vi "Init.vi"(5 "PathControl.lvclass":refnum<class "PathControl.lvclass">, 6 "Environmental classes":refnum<class "Instrument.lvclass">[](array[class]), 7 "XML Handler.lvclass":refnum<class "XML Handler.lvclass">, 8 "error in (no error)":errorcluster, 9 "Instrumentes to Use":T1(array[cluster]), 10 "Device.lvclass":refnum<class "Device.lvclass">, 11 "MCCW ACLR in":refnum<class "MCCW ACLR.lvclass">) -> (0 "error out":errorcluster, 3 "MCCW ACLR out":refnum<class "MCCW ACLR.lvclass">)   [LabVIEW 2020, in "MCCW ACLR.lvclass"]
doc: "Initializes the measurement.\nThis verifies that the instruments are present and adds them into the class data.\nIs also adds the xml handler into the class data."
uses:
  MCCW ACLR.lvclass
  C:/Sandbox/Git_Sandbox/WiSpry Test Framework source code (LV20)/WiSpry Test Framework/Measurements/Measurement.lvclass
  Devices/Device.lvclass
  Instruments/Instrument.lvclass
  XML Handler/XML Handler.lvclass
  Path Control/PathControl.lvclass
  Controls/Init States.ctl
  Instruments/Vector Signal Generator/Vector Signal Generator.lvclass
  Instruments/Spectrum Analyzer/Spectrum Analyzer.lvclass
  MCCW ACLR.lvclass/MCCW ACLR.ctl
  Measurement.lvclass/Measurement.ctl
  Devices/Controls/Change setting mode enum.ctl
  Path Control/Measurements Specific Paths.ctl
  Measurement.lvclass
  Devices/PIC-device/PIC-Device.lvclass
panel:
  out "Current State":string
  out "Initializing MCCW ACLR Measurement":u8(slide) scale=0.0..100.0
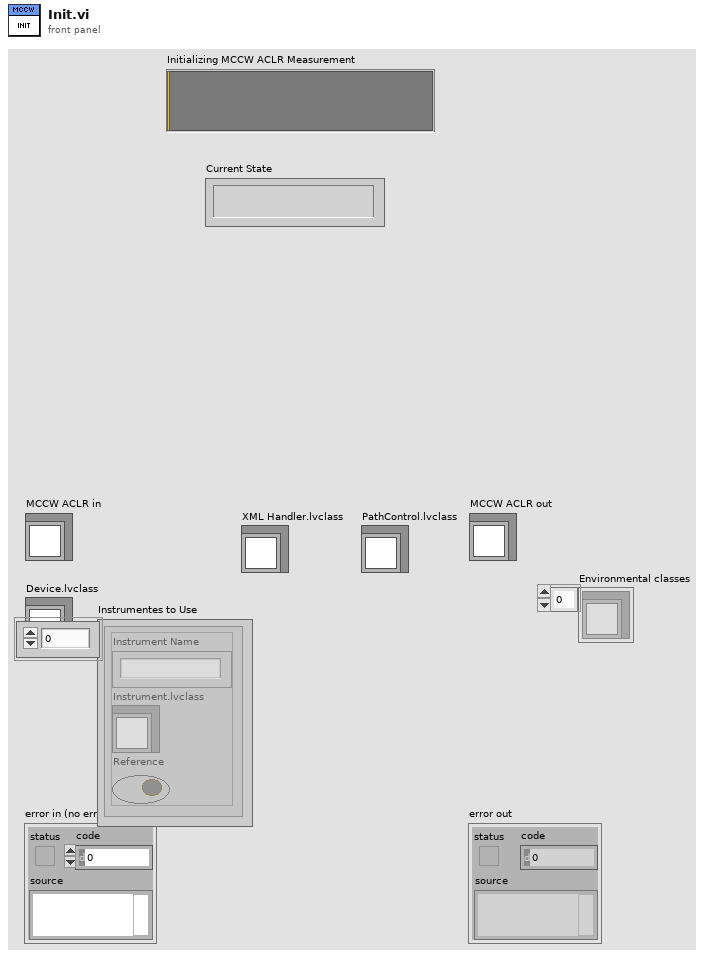
[diagram p1: front panel]
types:
  T1 = cluster{"Instrument Name":string, "Instrument.lvclass":refnum<class "Instrument.lvclass">, "Reference":bool}[]
  T2 = typedef "Measurement.lvclass/Init States.ctl" = enum16{"Verify instruments", "Init Parameters", "Init Instruments", "Add Device", "Init Device", "Create test in XML", "Set path", "Done"}
  T3 = cluster{"List":dbl[], "Index":i32, "Last":bool, "BW [MHz]":dbl}
  T4 = cluster{"Number of Measurements":u32, "Current Measurement":u32, "Last":bool}
  T5 = enum16{"ACLR Configuration", "Reference Level", "Both"}
  T6 = typedef "PIC-Device.lvclass/Change setting mode enum.ctl" = enum16{"Init", "Next", "Reset"}
  T7 = typedef "PathControl.lvclass/Measurements Specific Paths.ctl" = enum16{"No calibration", "Harmonics", "IMD", "S Parameter", "AM-AM", "MCCW-ACLR", "DC", "LCR", "Power Meter GUI", "RF Power"}
  T8 = typedef "MCCW ACLR.lvclass/ACLR configuration.ctl" = cluster{"Frequency":cluster{"Cluster ":cluster{"From":dbl, "To":dbl, "Step":dbl}, "Array":dbl[], "Use Array":bool}, "Power":cluster{"Cluster ":cluster{"From":dbl, "To":dbl, "Step":dbl}, "Array":dbl[], "Use Array":bool}, "Carriers":cluster{"Cluster ":cluster{"From":dbl, "To":dbl, "Step":dbl}, "Array":dbl[], "Use Array":bool}, "Phase Value":dbl, "Number of Measurements":u32, "Use random phase":bool, "Signal BW [MHz] ":dbl}
  T9 = cluster{"Cluster ":cluster{"From":dbl, "To":dbl, "Step":dbl}, "Array":dbl[], "Use Array":bool}
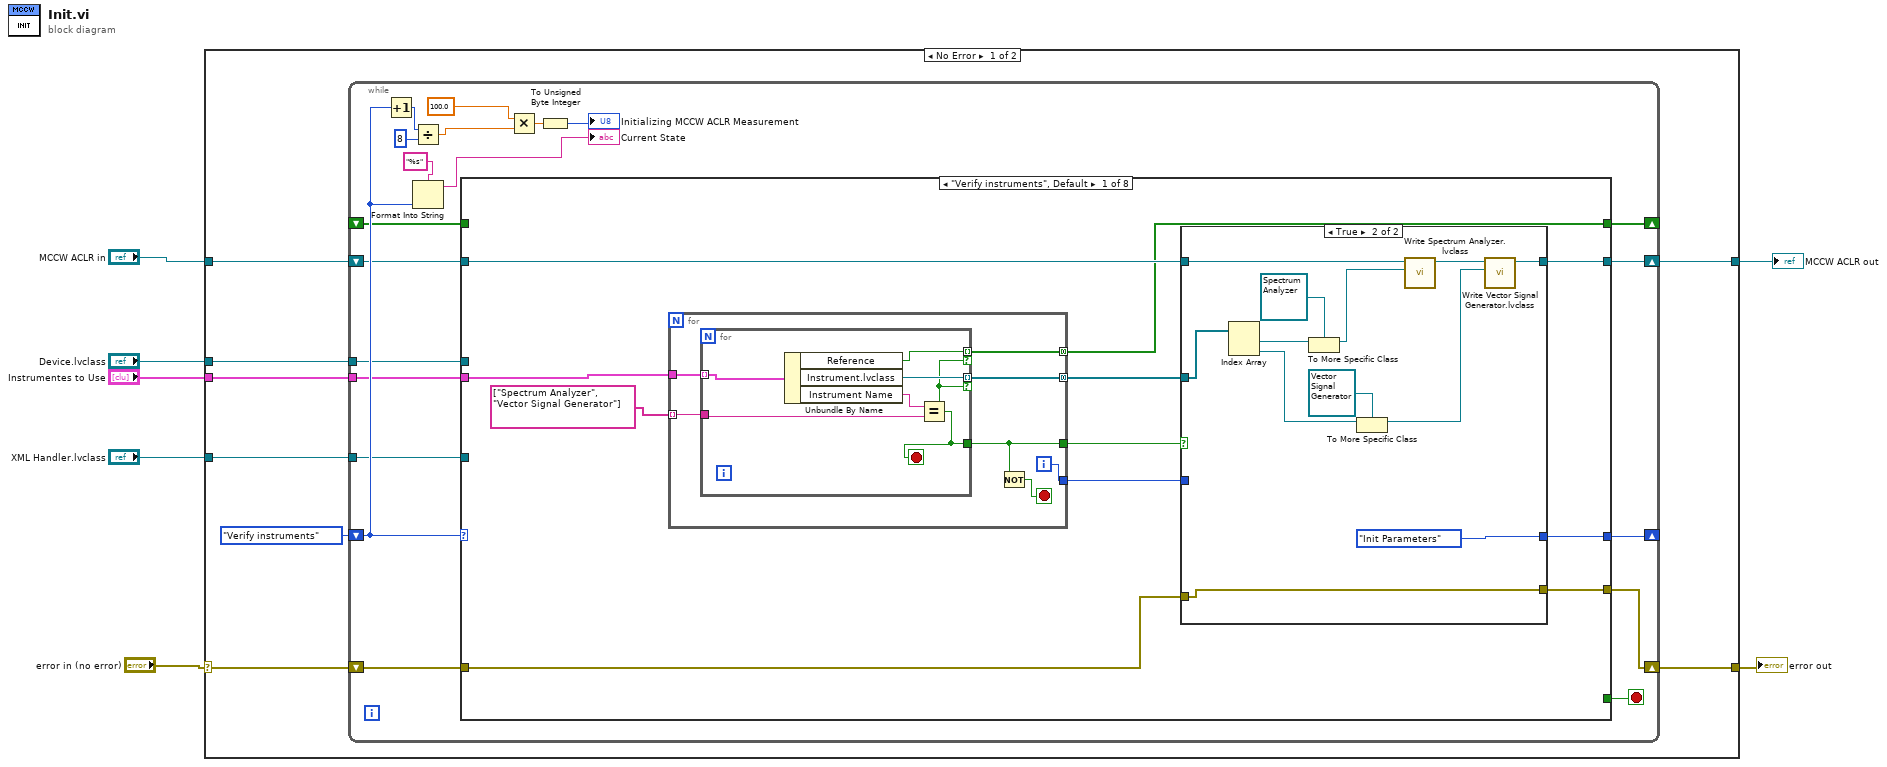
[diagram p0: block diagram]
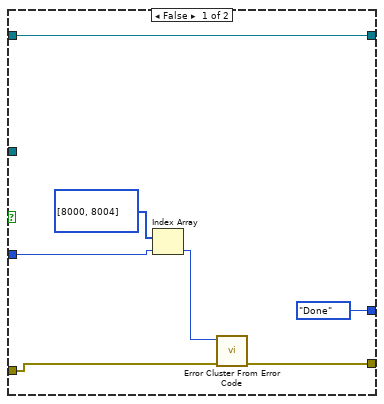
[diagram p2: hidden frame]
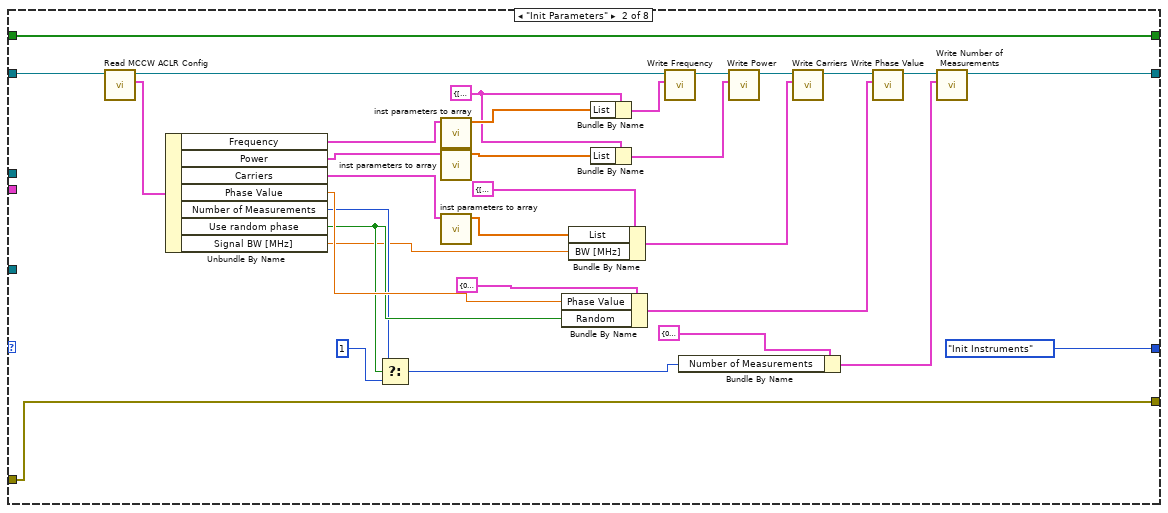
[diagram p3: hidden frame]
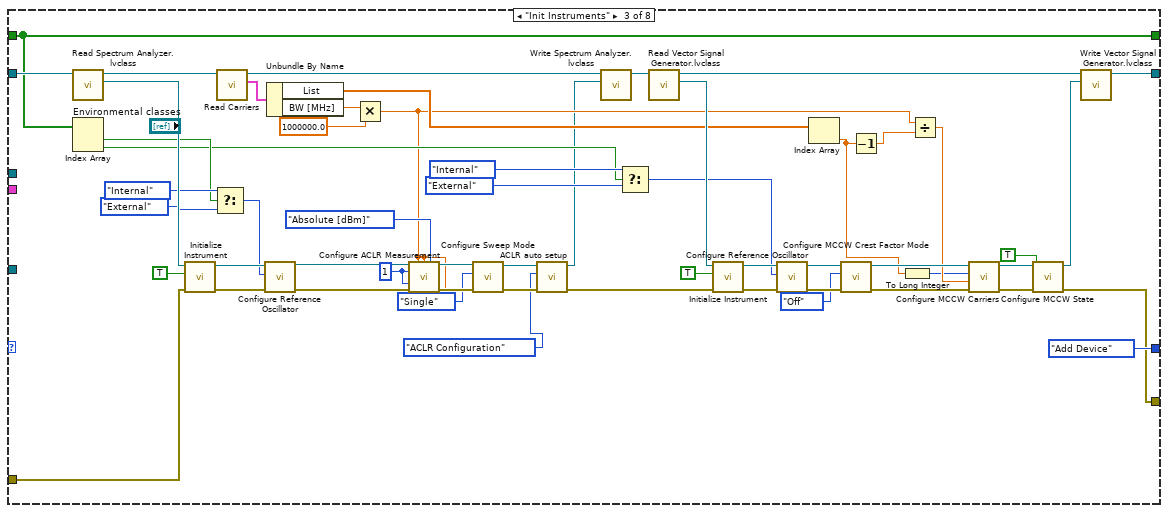
[diagram p4: hidden frame]
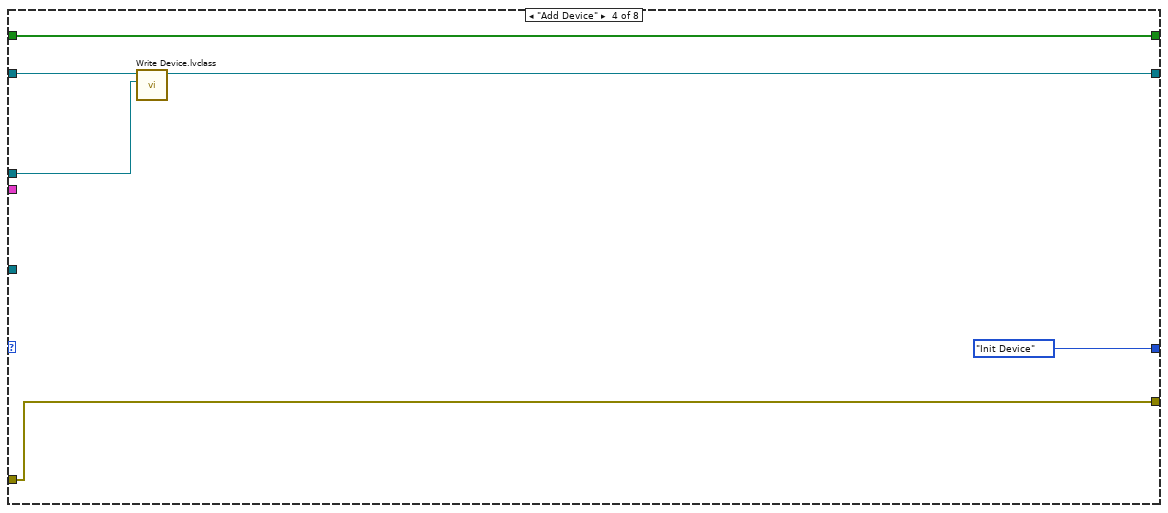
[diagram p5: hidden frame]
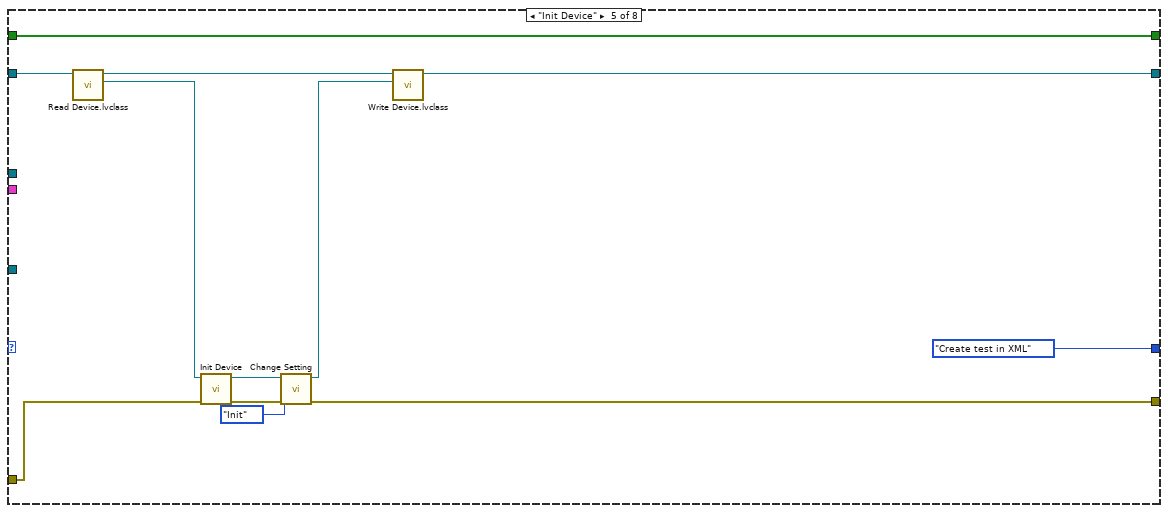
[diagram p6: hidden frame]
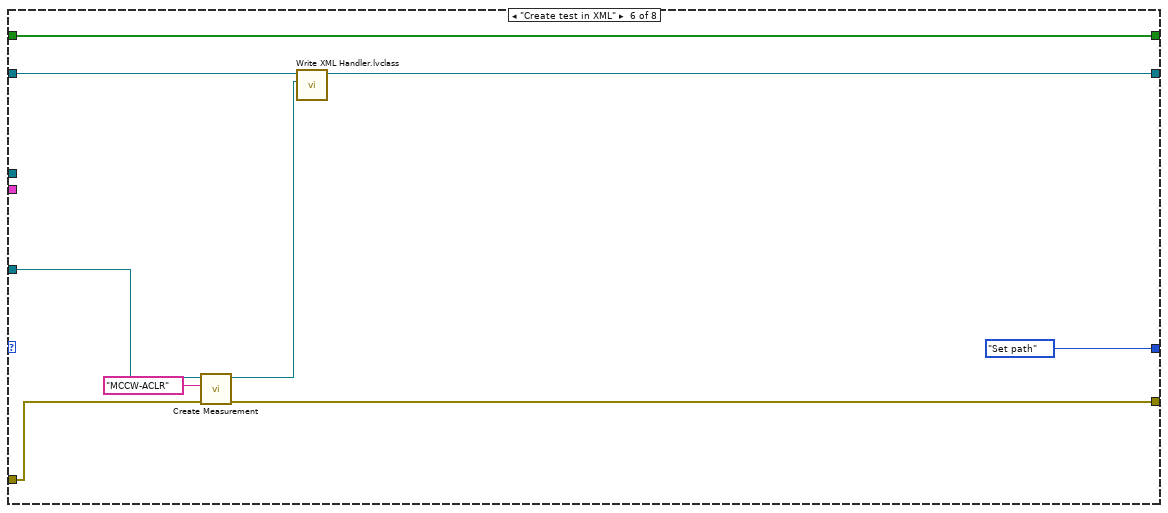
[diagram p7: hidden frame]
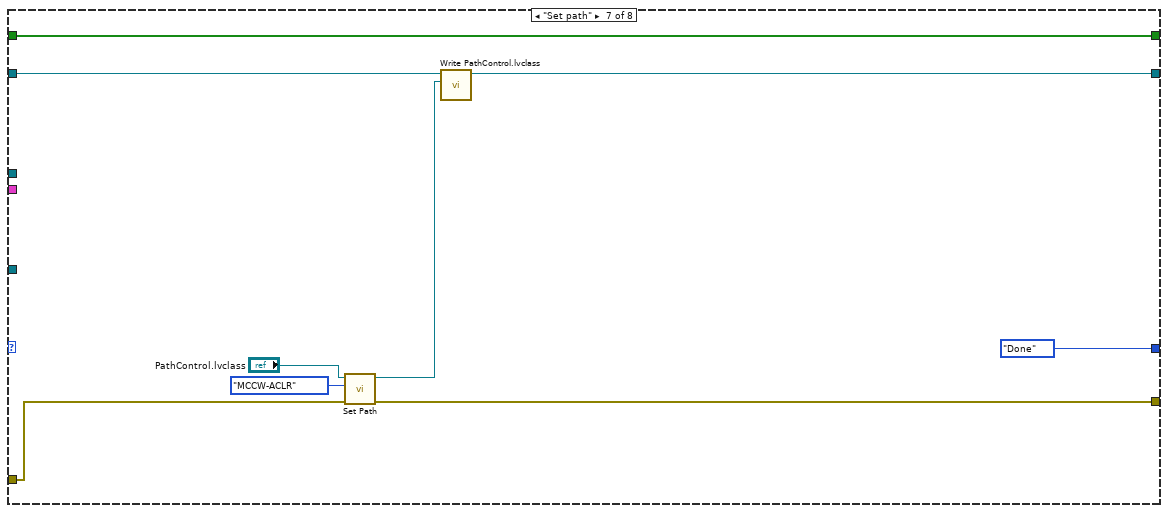
[diagram p8: hidden frame]
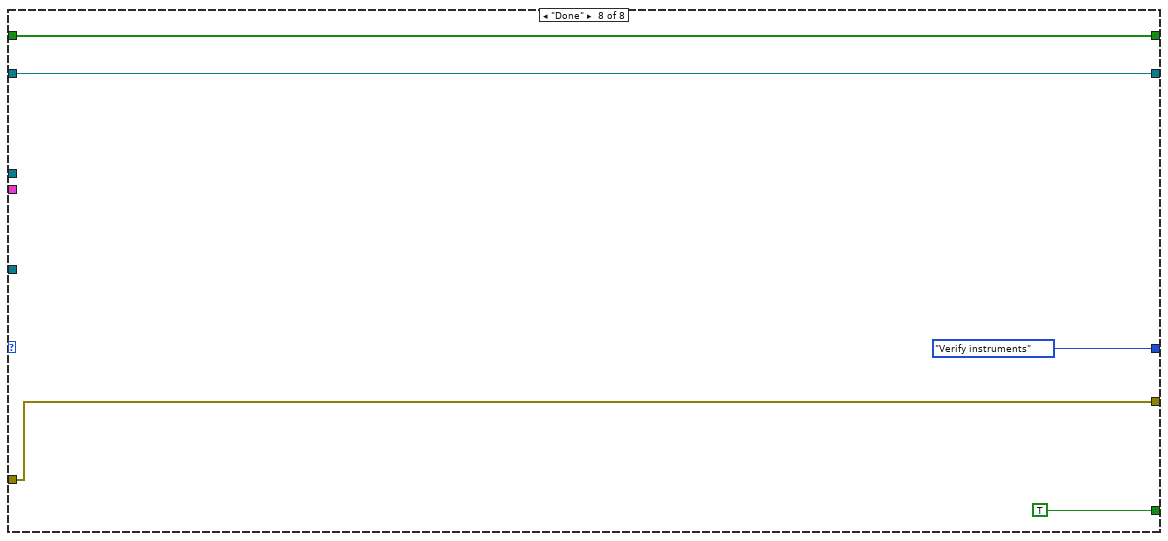
[diagram p9: hidden frame]
diagram:
  n1 = case shown="No Error" "error in (no error)" {
    selector: "error in (no error)" -> [w14 w208]
    tunnel: "MCCW ACLR in" -> [w13 w209]
    tunnel: "Device.lvclass" -> [w12 _]
    tunnel: "Instrumentes to Use" -> [w11 _]
    tunnel: "XML Handler.lvclass" -> [w10 _]
    tunnel: [w9 w208] -> w2
    tunnel: [w8 w209] -> w1
    frame No Error {
      n2 = while {
        shift-right: [w21] -> _
        shift-left: Init_States."Verify instruments" ("Init States") -> [w27]
        shift-right: [w20] -> w9
        shift-left: w14 -> [w23]
        tunnel: w12 -> [w25]
        tunnel: w11 -> [w26]
        tunnel: w10 -> [w17]
        shift-right: [w22] -> w8
        shift-left: w13 -> [w24]
        shift-right: [w19] -> _
        shift-left: _ -> [w18]
        stop <- w16 stop-if-true
        n3 = Increment(x=w27) -> (x+1=w35:T2)
        n4 = Divide(x=w35, y=8) -> (x/y=w32:dbl)
        n5 = Format Into String(format string="%s", w27) -> (resulting string=→"Current State":string)  [unwired: 2 in, 1 out]
        n6 = case shown="\"Verify instruments\", Default" w27 {
          tunnel: w26 -> [w46 _ _ _ _ _ _ _]
          tunnel: w25 -> [_ _ _ w171 _ _ _ _]
          tunnel: w24 -> [w43 w110 w166 w172 w183 w188 w197 w205]
          tunnel: w23 -> [w39 w84 w163 w168 w182 w192 w201 w207]
          tunnel: [w41 w89 w117 w170 w174 w186 w195 w205] -> w22
          tunnel: [w40 Init_States."Init Instruments" ("Init States") Init_States."Add Device" ("Init States") Init_States."Init Device" ("Init States") Init_States."Create test in XML" ("Init States") Init_States."Set path" ("Init States") Init_States."Done" ("Init States") Init_States."Verify instruments" ("Init States")] -> w21
          tunnel: [w37 w84 w116 w168 w175 w191 w200 w207] -> w20
          tunnel: [w36 w82 w165 w169 w184 w193 w202 w206] -> w19
          tunnel: w18 -> [_ w82 w165 w169 w184 w193 w202 w206]
          tunnel: w17 -> [_ _ _ _ _ w190 _ _]
          tunnel: [_ _ _ _ _ _ _ TRUE] -> w16
          frame "Verify instruments", Default {
            n7 = for {
              tunnel: w46 -> [w72]
              tunnel: string[] ["Spectrum Analyzer", "Vector Signal Generator"] -> [w68] mode=indexing
              tunnel: [w71] -> w42 mode=concatenating
              tunnel: [w70] -> w44
              tunnel: [w67] -> w38
              tunnel: [w66] -> w36 mode=concatenating
              i -> [w67]
              stop <- w69 stop-if-true
              n8 = for {
                tunnel: w72 -> [w78] mode=indexing
                tunnel: w68 -> [w76]
                tunnel: [w75] -> w71 mode=indexing if=w73
                tunnel: [w73] -> w70
                tunnel: [w74] -> w66 mode=indexing if=w73
                stop <- w73 stop-if-true
                n9 = Unbundle By Name(w78) -> ("Reference"=w74:bool, "Instrument.lvclass"=w75:refnum<class "Instrument.lvclass">, "Instrument Name"=w77:string)
                n10 = Equal?(x=w77, y=w76) -> (x = y?=w73:bool)
              }
              n11 = Not(x=w70) -> (.not. x?=w69:bool)
            }
            n12 = case shown="True" w44 {
              tunnel: w43 -> [w47 w65]
              tunnel: w42 -> [_ w63]
              tunnel: [w47 w56] -> w41
              tunnel: [Init_States."Done" ("Init States") Init_States."Init Parameters" ("Init States")] -> w40
              tunnel: w39 -> [w52 w54]
              tunnel: w38 -> [w50 _]
              tunnel: [w48 w54] -> w37
              frame False {
                n13 = Index Array(array=i32[] [8000, 8004], index=w50) -> (element=w49:i32)
                n14 = call <vilib>:"Error Cluster From Error Code.vi"("error in (no error)"=w52, "error code (0)"=w49) -> ("error out"=w48:errorcluster)  [unwired: 7 in]
              }
              frame True {
                n15 = Index Array(array=w63) -> (element #1=w62:refnum<class "Instrument.lvclass">, element #2=w58:refnum<class "Instrument.lvclass">)  [unwired: 2 in]
                n16 = To More Specific Class(target class=refnum<class "Spectrum Analyzer.lvclass"> refnum ("Spectrum Analyzer.lvclass"), reference=w62) -> (specific class reference=w60:refnum<class "Spectrum Analyzer.lvclass">)  [unwired: 1 in, 1 out]
                n17 = To More Specific Class(target class=refnum<class "Vector Signal Generator.lvclass"> refnum ("Vector Signal Generator.lvclass"), reference=w58) -> (specific class reference=w57:refnum<class "Vector Signal Generator.lvclass">)  [unwired: 1 in, 1 out]
                n18 = call "Write Spectrum Analyzer.lvclass.vi"("Spectrum Analyzer.lvclass"=w60, "MCCW ACLR in"=w65) -> ("MCCW ACLR out"=w64:refnum<class "MCCW ACLR.lvclass">)  [unwired: 9 in]
                n19 = call "Write Vector Signal Generator.lvclass.vi"("Vector Signal Generator.lvclass"=w57, "MCCW ACLR in"=w64) -> ("MCCW ACLR out"=w56:refnum<class "MCCW ACLR.lvclass">)  [unwired: 9 in]
              }
            }
          }
          frame "Init Parameters" {
            w102 = cluster{"List":dbl[], "Index":i32, "Last":bool} {"List"=[], "Index"=0, "Last"=FALSE} ("Frequency")
            n20 = call "Read MCCW ACLR Config.vi"("MCCW ACLR in"=w110) -> ("MCCW ACLR Config"=w109:T8, "MCCW ACLR out"=w105:refnum<class "MCCW ACLR.lvclass">)  [unwired: 9 in]
            n21 = Unbundle By Name(w109) -> ("Frequency"=w108:T9, "Power"=w107:T9, "Carriers"=w106:T9, "Phase Value"=w94:dbl, "Number of Measurements"=w86:u32, "Use random phase"=w87:bool, "Signal BW [MHz]"=w80:dbl)
            n22 = Select(t=w86, s=w87, f=u32 1) -> (s? t:f=w88:u32)
            n23 = call "inst parameters to array.vi"("Input"=w108) -> ("Array"=w104:dbl[])  [unwired: 10 in]
            n24 = call "inst parameters to array.vi"("Input"=w107) -> ("Array"=w101:dbl[])  [unwired: 10 in]
            n25 = call "inst parameters to array.vi"("Input"=w106) -> ("Array"=w100:dbl[])  [unwired: 10 in]
            n26 = Bundle By Name(cluster=cluster{"Phase Value":dbl, "Random":bool} {"Phase Value"=0.0, "Random"=FALSE} ("Phase Value"), "Phase Value"=w94, "Random"=w87) -> (w93:cluster{"Phase Value":dbl, "Random":bool})
            n27 = Bundle By Name(cluster=T3 {"List"=[], "Index"=0, "Last"=FALSE, "BW [MHz]"=0.0} ("Carriers"), "List"=w100, "BW [MHz]"=w80) -> (w79:T3)
            n28 = Bundle By Name(cluster=w102, "List"=w104) -> (w103:cluster{"List":dbl[], "Index":i32, "Last":bool})
            n29 = Bundle By Name(cluster=w102, "List"=w101) -> (w98:cluster{"List":dbl[], "Index":i32, "Last":bool})
            n30 = call "Write Frequency.vi"("Frequency"=w103, "MCCW ACLR in"=w105) -> ("MCCW ACLR out"=w99:refnum<class "MCCW ACLR.lvclass">)  [unwired: 9 in]
            n31 = Bundle By Name(cluster=T4 {"Number of Measurements"=0, "Current Measurement"=0, "Last"=FALSE} ("Number of Measurements"), "Number of Measurements"=w88) -> (w90:T4)
            n32 = call "Write Power.vi"("Power"=w98, "MCCW ACLR in"=w99) -> ("MCCW ACLR out"=w97:refnum<class "MCCW ACLR.lvclass">)  [unwired: 9 in]
            n33 = call "Write Carriers.vi"("Carriers"=w79, "MCCW ACLR in"=w97) -> ("MCCW ACLR out"=w96:refnum<class "MCCW ACLR.lvclass">)  [unwired: 9 in]
            n34 = call "Write Phase Value.vi"("Phase Value"=w93, "MCCW ACLR in"=w96) -> ("MCCW ACLR out"=w92:refnum<class "MCCW ACLR.lvclass">)  [unwired: 9 in]
            n35 = call "Write Number of Measurements.vi"("Number of Measurements"=w90, "MCCW ACLR in"=w92) -> ("MCCW ACLR out"=w89:refnum<class "MCCW ACLR.lvclass">)  [unwired: 9 in]
          }
          frame "Init Instruments" {
            w153 = 1 ("TX Channels")
            n36 = call "Read Spectrum Analyzer.lvclass.vi"("MCCW ACLR in"=w166) -> ("Spectrum Analyzer.lvclass"=w164:refnum<class "Spectrum Analyzer.lvclass">, "MCCW ACLR out"=w152:refnum<class "MCCW ACLR.lvclass">)  [unwired: 9 in]
            n37 = Index Array(array=w165) -> (element #1=w158:bool, element #2=w137:bool)  [unwired: 2 in]
            n38 = call-dynamic "Initialize Instrument.vi"("error in (no error)"=w163, "Reset"=TRUE, "Instrument in"=w164) -> ("error out"=w161:errorcluster, "Instrument out"=w160:refnum<class "Spectrum Analyzer.lvclass">)  [unwired: 7 in]
            n39 = Select(t=enum16{"Internal", "External"}."Internal" ("Reference Oscillator (Internal)"), s=w158, f=enum16{"Internal", "External"}."External") -> (s? t:f=w156:enum16{"Internal", "External"})
            n40 = call "Read Carriers.vi"("MCCW ACLR in"=w152) -> ("Carriers"=w151:T3, "MCCW ACLR out"=w143:refnum<class "MCCW ACLR.lvclass">)  [unwired: 9 in]
            n41 = call-dynamic "Configure Reference Oscillator.vi"("error in (no error)"=w161, "Reference Oscillator (Internal)"=w156, "Spectrum Analyzer in"=w160) -> ("error out"=w155:errorcluster, "Spectrum Analyzer out"=w154:refnum<class "Spectrum Analyzer.lvclass">)  [unwired: 7 in]
            n42 = Unbundle By Name(w151) -> ("List"=w129:dbl[], "BW [MHz]"=w150:dbl)
            n43 = Multiply(x=w150, y=1000000.0) -> (x*y=w126:dbl)
            n44 = call-dynamic "Configure ACLR Measurement.vi"("Spectrum Analyzer in"=w154, "TX Bandwidth [Hz]"=w126, "TX Spacing [Hz]"=w126, "ALCR Type"=enum16{"Relative [dBc]", "Absolute [dBm]"}."Absolute [dBm]", "TX Channels"=w153, "Adj Channels"=w153, "error in (no error)"=w155, "Adj Bandwidth [Hz]"=w126, "Adj Spacing [Hz]"=w126) -> ("Spectrum Analyzer out"=w146:refnum<class "Spectrum Analyzer.lvclass">, "error out"=w147:errorcluster)  [unwired: 5 in]
            n45 = call-dynamic "Configure Sweep Mode.vi"("error in (no error)"=w147, "Sweep Mode"=enum16{"Continuous", "Single"}."Single", "Spectrum Analyzer in"=w146) -> ("error out"=w115:errorcluster, "Spectrum Analyzer out"=w114:refnum<class "Spectrum Analyzer.lvclass">)  [unwired: 7 in]
            n46 = call-dynamic "ACLR auto setup.vi"("error in (no error)"=w115, "Setup"=T5."ACLR Configuration", "Spectrum Analyzer in"=w114) -> ("error out"=w112:errorcluster, "Spectrum Analyzer out"=w113:refnum<class "Spectrum Analyzer.lvclass">)  [unwired: 7 in]
            n47 = call "Write Spectrum Analyzer.lvclass.vi"("Spectrum Analyzer.lvclass"=w113, "MCCW ACLR in"=w143) -> ("MCCW ACLR out"=w142:refnum<class "MCCW ACLR.lvclass">)  [unwired: 9 in]
            n48 = Select(t=enum16{"Internal", "External"}."Internal" ("Reference Oscillator (Internal)"), s=w137, f=enum16{"Internal", "External"}."External") -> (s? t:f=w136:enum16{"Internal", "External"})
            n49 = call "Read Vector Signal Generator.lvclass.vi"("MCCW ACLR in"=w142) -> ("Vector Signal Generator.lvclass"=w141:refnum<class "Vector Signal Generator.lvclass">, "MCCW ACLR out"=w119:refnum<class "MCCW ACLR.lvclass">)  [unwired: 9 in]
            n50 = call-dynamic "Initialize Instrument.vi"("error in (no error)"=w112, "Reset"=TRUE, "Instrument in"=w141) -> ("error out"=w135:errorcluster, "Instrument out"=w140:refnum<class "Vector Signal Generator.lvclass">)  [unwired: 7 in]
            n51 = call-dynamic "Configure Reference Oscillator.vi"("error in (no error)"=w135, "Reference Mode"=w136, "Signal Generator in"=w140) -> ("error out"=w134:errorcluster, "Signal Generator out"=w133:refnum<class "Vector Signal Generator.lvclass">)  [unwired: 7 in]
            n52 = Index Array(array=w129) -> (element=w128:dbl)  [unwired: 1 in]
            n53 = call-dynamic "Configure MCCW Crest Factor Mode.vi"("error in (no error)"=w134, "Crest factor mode"=enum16{"Off", "Chirp", "Slow"}."Off", "Vector Signal Generator in"=w133) -> ("error out"=w131:errorcluster, "Vector Signal Generator out"=w130:refnum<class "Vector Signal Generator.lvclass">)  [unwired: 7 in]
            n54 = Decrement(x=w128) -> (x-1=w127:dbl)
            n55 = To Long Integer(number=w128) -> (32bit integer=w124:i32)
            n56 = Divide(x=w126, y=w127) -> (x/y=w125:dbl)
            n57 = call-dynamic "Configure MCCW Carriers.vi"("error in (no error)"=w131, "MCCW Carrier spacing [Hz]"=w125, "MCCW Carriers"=w124, "Vector Signal Generator in"=w130) -> ("error out"=w123:errorcluster, "Vector Signal Generator out"=w122:refnum<class "Vector Signal Generator.lvclass">)  [unwired: 6 in]
            n58 = call-dynamic "Configure MCCW State.vi"("error in (no error)"=w123, "State"=TRUE, "Vector Signal Generator in"=w122) -> ("error out"=w116:errorcluster, "Vector Signal Generator out"=w118:refnum<class "Vector Signal Generator.lvclass">)  [unwired: 7 in]
            n59 = call "Write Vector Signal Generator.lvclass.vi"("Vector Signal Generator.lvclass"=w118, "MCCW ACLR in"=w119) -> ("MCCW ACLR out"=w117:refnum<class "MCCW ACLR.lvclass">)  [unwired: 9 in]
          }
          frame "Add Device" {
            n60 = call "Write Device.lvclass.vi"("Device.lvclass"=w171, "Measurements in"=w172) -> ("Measurements out"=w170:refnum<class "MCCW ACLR.lvclass">)  [unwired: 9 in]
          }
          frame "Init Device" {
            n61 = call "Read Device.lvclass.vi"("Measurements in"=w183) -> ("Device.lvclass"=w181:refnum<class "Device.lvclass">, "Measurements out"=w177:refnum<class "MCCW ACLR.lvclass">)  [unwired: 9 in]
            n62 = call-dynamic "Init Device.vi"("error in (no error)"=w182, "Device in"=w181) -> ("error out"=w180:errorcluster, "Device out"=w179:refnum<class "Device.lvclass">)  [unwired: 8 in]
            n63 = call-dynamic "Change Setting.vi"("error in (no error)"=w180, "Change setting mode"=Change_setting_mode_enum."Init", "Device in"=w179) -> ("error out"=w175:errorcluster, "Device out"=w176:refnum<class "Device.lvclass">)  [unwired: 5 in, 2 out]
            n64 = call "Write Device.lvclass.vi"("Device.lvclass"=w176, "Measurements in"=w177) -> ("Measurements out"=w174:refnum<class "MCCW ACLR.lvclass">)  [unwired: 9 in]
          }
          frame "Create test in XML" {
            n65 = call "Create Measurement.vi"("error in (no error)"=w192, "Measurement Name"="MCCW-ACLR", "XML Handler in"=w190) -> ("error out"=w191:errorcluster, "XML Handler out"=w187:refnum<class "XML Handler.lvclass">)  [unwired: 7 in]
            n66 = call "Write XML Handler.lvclass.vi"("XML Handler.lvclass"=w187, "Measurements in"=w188) -> ("Measurements out"=w186:refnum<class "MCCW ACLR.lvclass">)  [unwired: 9 in]
          }
          frame "Set path" {
            n67 = call "Set Path.vi"("error in (no error)"=w201, "Measurement specfic paths"=Measurements_Specific_Paths."MCCW-ACLR", "PathControl in"="PathControl.lvclass") -> ("error out"=w200:errorcluster, "PathControl out"=w196:refnum<class "PathControl.lvclass">)  [unwired: 7 in]
            n68 = call "Write PathControl.lvclass.vi"("PathControl.lvclass"=w196, "Measurements in"=w197) -> ("Measurements out"=w195:refnum<class "MCCW ACLR.lvclass">)  [unwired: 9 in]
          }
          frame "Done" {
          }
        }
        n69 = Multiply(x=100.0 ("y"), y=w32) -> (x*y=w34:dbl)
        n70 = To Unsigned Byte Integer(number=w34) -> (unsigned 8bit integer=→"Initializing MCCW ACLR Measurement":u8)
      }
    }
    frame Error {
    }
  }
  "error out" <- w2
  "MCCW ACLR out" <- w1
